vi "RemoveBus.vi"(7 "Remove All? (F)":bool, 8 "ErrorArray In":errorcluster[](array[cluster])) -> (0 "ErrorArray Out":errorcluster[](array[cluster]))   [LabVIEW 2017, in "Bus_class.lvlib" / "Bus.lvclass"]
uses:
  Bus.lvclass
  <userlib>/NIST/ModuleAdminLib/ModuleAdmin/ModuleAdmin.lvclass
  Bus.lvclass/Bus.ctl
  <vilib>/Utility/miscctls.llb/LVStringsAndValuesArrayTypeDef_U8.ctl
  Accessors/Read OutputToFileModuleID.vi
  <vilib>/Utility/error.llb/Error Cluster From Error Code.vi
  <vilib>/ErrorRing/Error Ring.xnode
  Modules/EventModule/EventModule.lvlib
  <userlib>/NIST/NISTErrorLib/NISTErrorLib.lvlib
  Framework.lvlib
  Modules/PmuImpairModule/PmuImpairModule.lvlib
  Modules/NetworkImpairmentModule/NetworkImpairmentModule.lvlib
  Modules/FlagImpairModule/FlagImpairModule.lvlib
  Bus_class.lvlib
  Modules/OutputToFileModule/OutputToFileModule.lvlib
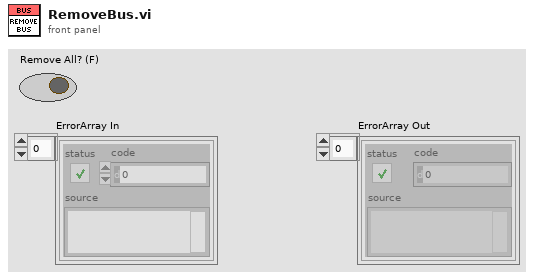
[diagram p1: front panel]
types:
  T1 = typedef "LVStringsAndValuesArrayTypeDef_U8.ctl" = cluster{"String":string, "Value":u8}[]
  T2 = typedef "Framework.lvlib/clFrontPanelControlRefs.ctl" = cluster{"TestFilePathRef":refnum<vi>, "BusNumberRef":refnum<vi>, "NumberOfBusesRef":refnum<vi>, "EvtTypeRef":refnum<vi>, "EvtParamsRef":refnum<vi>, "EvtConfigRef":refnum<vi>, "StartTimeRef":refnum<vi>, "EndTimeRef":refnum<vi>, "PmuImpairTypeRef":refnum<vi>, "PmuImpairParamsRef":refnum<vi>, "NetImpairParamsRef":refnum<vi>, "FlagImpairTypeRef":refnum<vi>, "FlagImpairParamsRef":refnum<vi>, "NetImpairTypeRef":refnum<vi>, "OutputFileType":refnum<vi>, "PmuImpairConfigRef":refnum<vi>, "AppTypeRef":refnum<vi>, "ScriptPathRef":refnum<vi>, "ShowPanels?":refnum<vi>}
  T3 = typedef "Framework.lvlib/clFrameworkData.ctl" = cluster{"EvtINIFilePaths":path[], "BusClassInstances":refnum<class "Bus.lvclass">[], "PmuImpairINIFilePaths":path[], "FlagImpairINIFilePaths":path[], "NetImpairINIFilePaths":path[], "OutputToFileINIFilePaths":path[], "AppINIFilePaths":path[], "AppModuleID":i32, "OutputToFileID":i32}
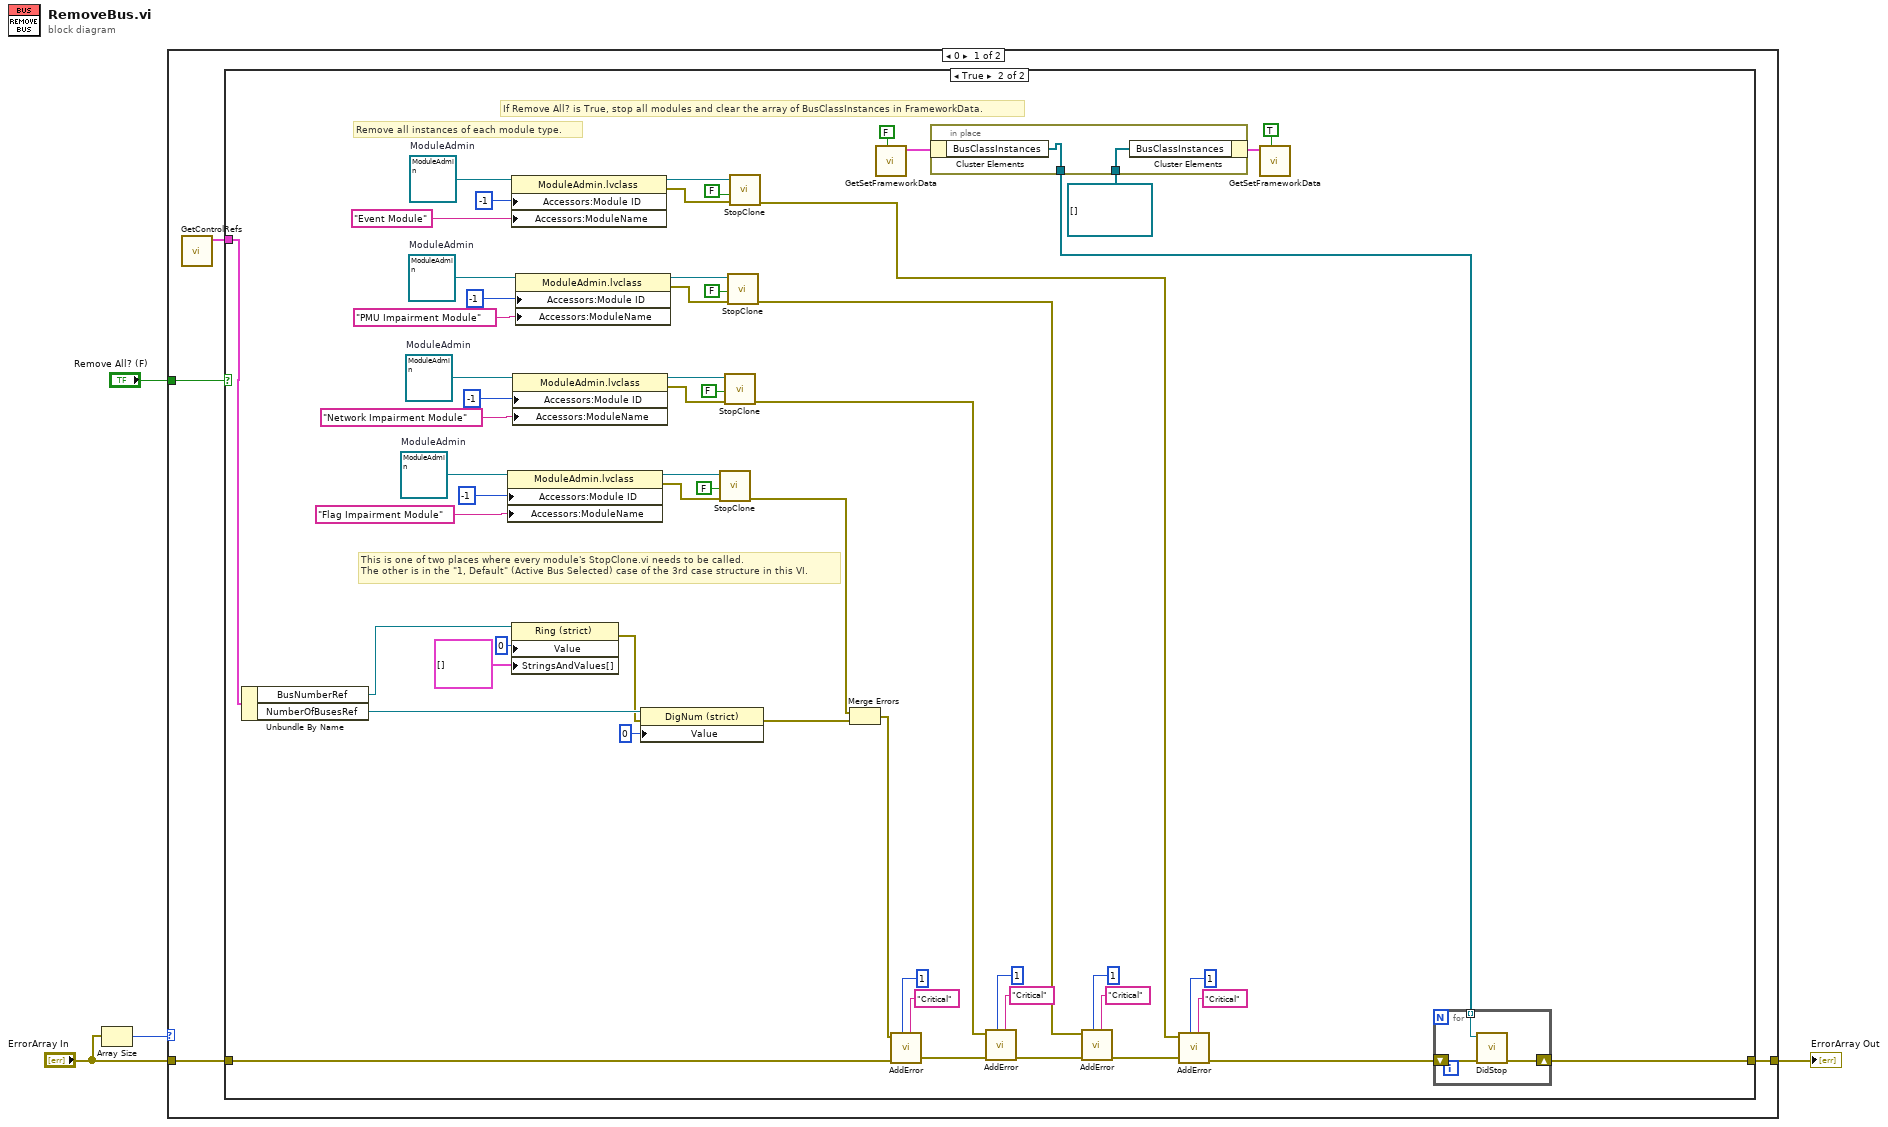
[diagram p0: block diagram]
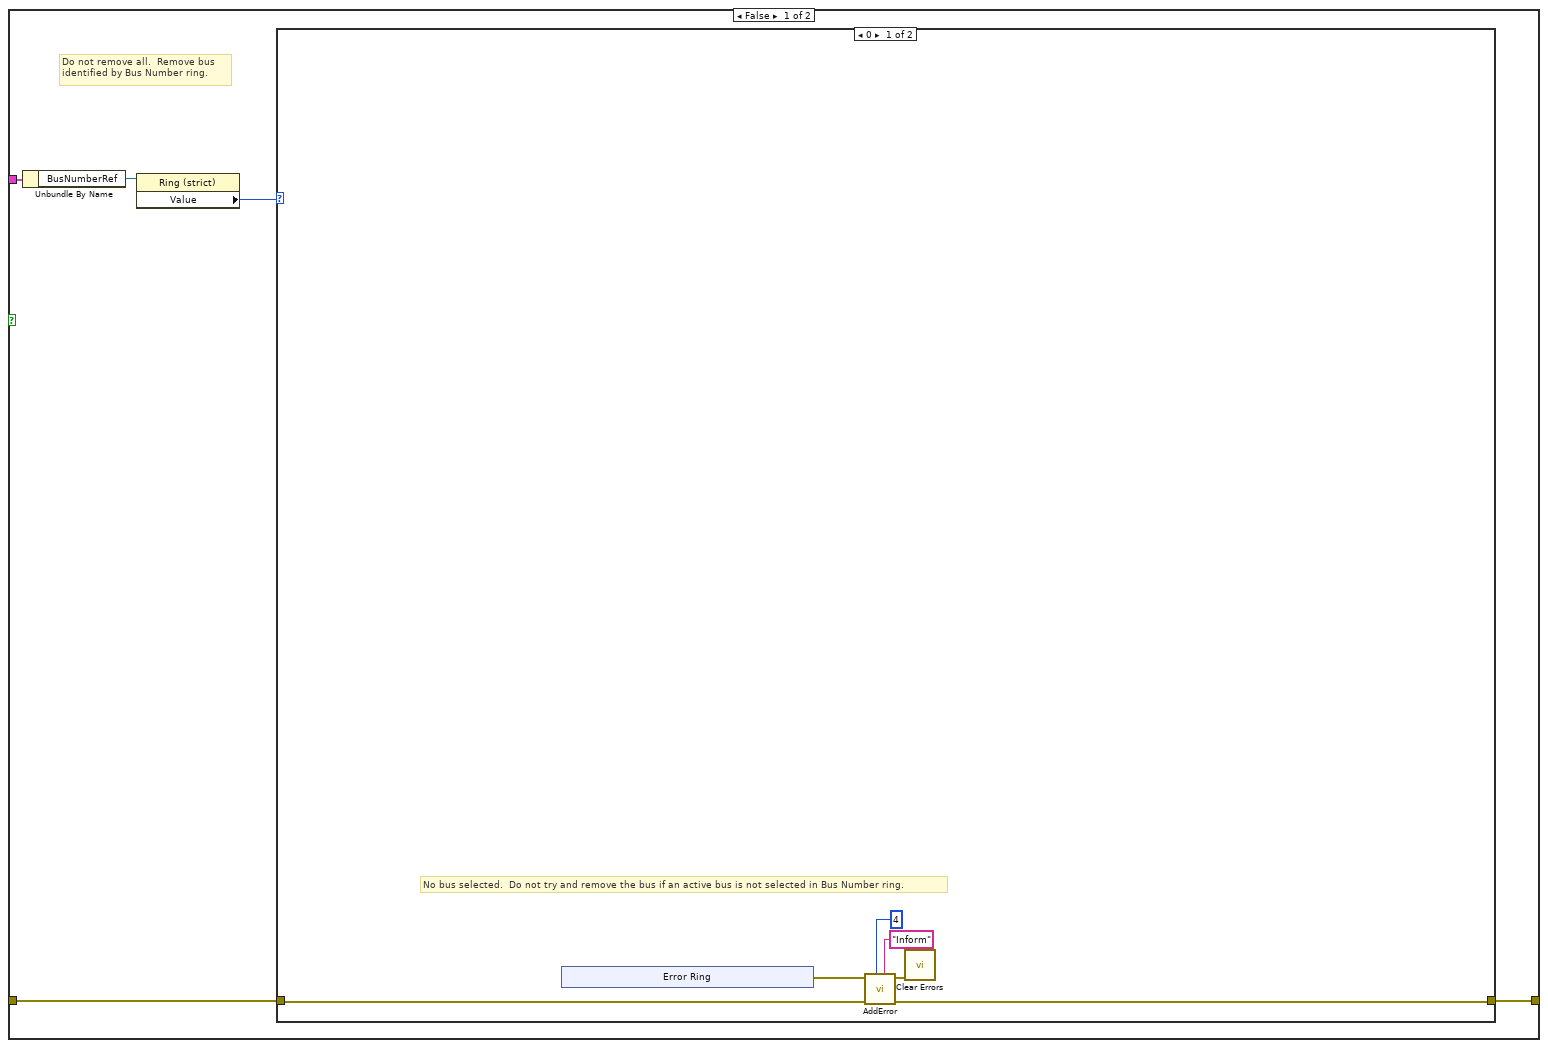
[diagram p2: hidden frame]
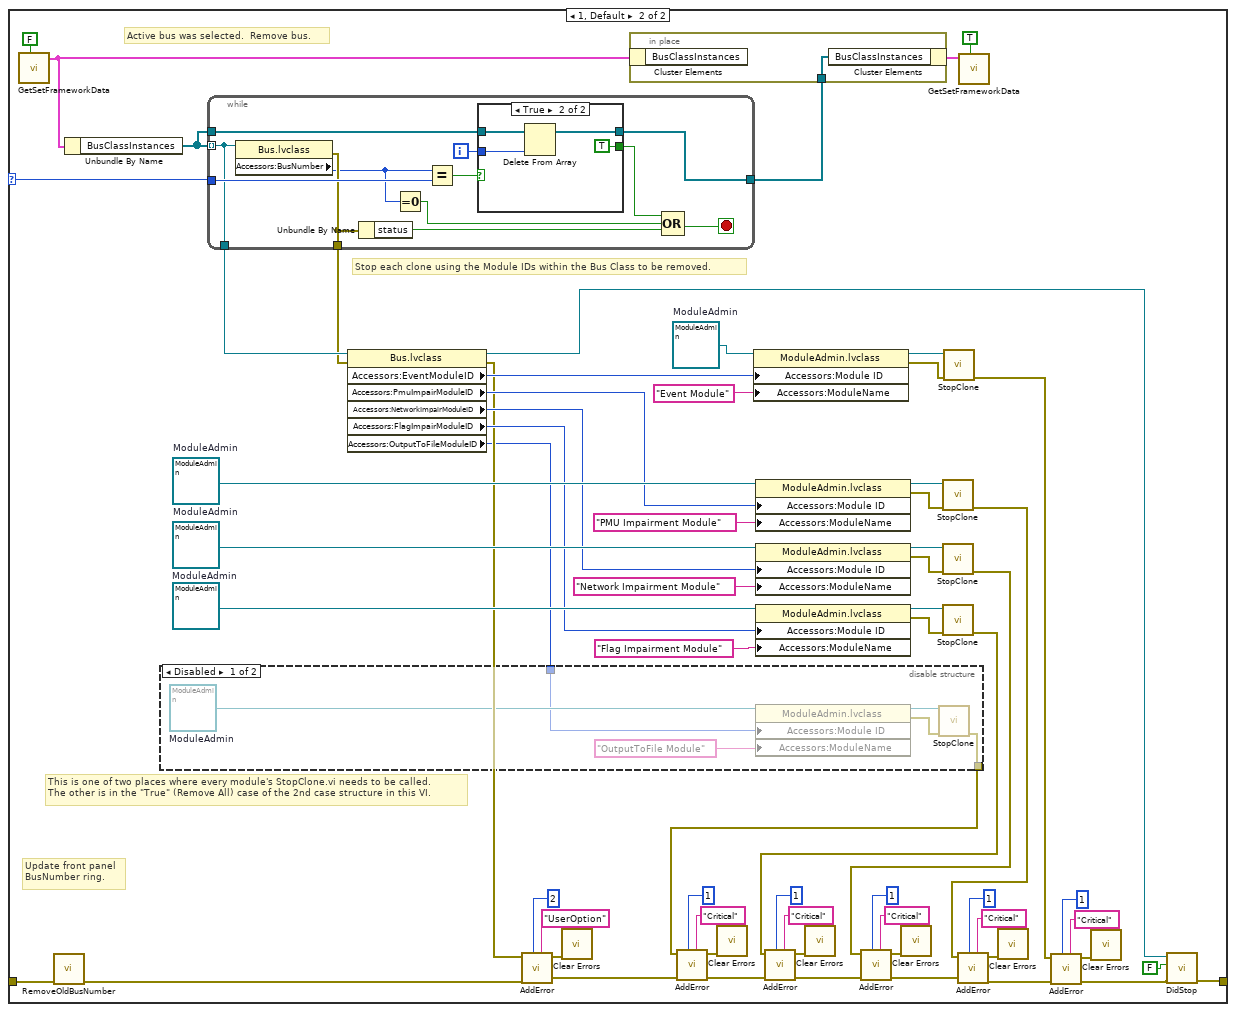
[diagram p3: hidden frame]
diagram:
  n1 = Array Size(array="ErrorArray In") -> (size(s)=w4:i32)
  n2 = case shown="0" w4 {
    tunnel: "ErrorArray In" -> [w7 w176]
    tunnel: [w8 w176] -> w2
    tunnel: "Remove All? (F)" -> [w6 _]
    frame 0 {
      n3 = call "GetControlRefs.vi"() -> ("clControlRefs Out"=w5:T2)  [unwired: 11 in]
      n4 = case shown="True" w6 {
        tunnel: [w13 w127] -> w8
        tunnel: w7 -> [w12 w124]
        tunnel: w5 -> [w9 w114]
        frame False {
          # "Do not remove all.  Remove bus\nidentified by Bus Number ring."
          n5 = Unbundle By Name(w9) -> ("BusNumberRef"=w11:refnum<vi>)
          n6 = property class="Ring (strict)"(reference=w11) -> ("Value"=w10:u8)  [unwired: 1 in, 2 out]
          n7 = case shown="0" w10 {
            selector: w10 -> [_ w77]
            tunnel: [w15 w34] -> w13
            tunnel: w12 -> [w16 w78]
            frame 0 {
              # "No bus selected.  Do not try and remove the bus if an active bus is not selected in Bus Number ring."
              n8 = xnode "Error Ring"() -> ("error out"=w14:errorcluster)
              n9 = call <userlib>:"AddError.vi"("Severity"="Inform" ("String"), "Priority"=u8 4, "ErrorArray"=w16, "error in (no error)"=w14) -> ("ErrorArray"=w15:errorcluster[], "error out"=w19:errorcluster)  [unwired: 6 in]
              n10 = call <vilib>:"Clear Errors.vi"("error in (no error)"=w19) -> ()  [unwired: 5 in, 2 out]
            }
            frame 1, Default {
              w59 = refnum<class "ModuleAdmin.lvclass"> refnum  # ModuleAdmin
              w65 = refnum<class "ModuleAdmin.lvclass"> refnum  # ModuleAdmin
              w69 = refnum<class "ModuleAdmin.lvclass"> refnum  # ModuleAdmin
              w72 = refnum<class "ModuleAdmin.lvclass"> refnum  # ModuleAdmin
              # "Update front panel\nBusNumber ring."
              # "This is one of two places where every module's StopClone.vi needs to be called.\nThe other is in the \"True\" (Remove All) case of the 2nd case structure in this VI."
              # "Stop each clone using the Module IDs within the Bus Class to be removed."
              # "Active bus was selected.  Remove bus."
              n11 = call "GetSetFrameworkData.vi"("Set (F)"=FALSE ("Set/Get")) -> ("clFrameworkData Out"=w85:T3)  [unwired: 10 in]
              n12 = call "RemoveOldBusNumber.vi"("ErrorArray In"=w78) -> ("ErrorArray Out"=w41:errorcluster[])  [unwired: 10 in]
              n13 = Unbundle By Name(w85) -> ("BusClassInstances"=w82:refnum<class "Bus.lvclass">[])
              n14 = while {
                tunnel: w77 -> [w106]
                tunnel: w82 -> [w102] mode=indexing
                tunnel: w82 -> [w105]
                tunnel: [w103] -> w81
                tunnel: [w102] -> w80
                tunnel: [w100] -> w79
                i -> [w104]
                stop <- w101 stop-if-true
                n15 = property class="Bus.lvclass"(reference=w102) -> (error out=w100:errorcluster, "Accessors:BusNumber"=w97:u8)  [unwired: 1 in, 1 out]
                n16 = Unbundle By Name(w100) -> ("status"=w99:bool)
                n17 = Equal To 0?(x=w97) -> (x = 0?=w96:bool)
                n18 = Equal?(x=w97, y=w106) -> (x = y?=w107:bool)
                n19 = case shown="True" w107 {
                  tunnel: w105 -> [w108 w112]
                  tunnel: w104 -> [_ w111]
                  tunnel: [_ TRUE] -> w98
                  tunnel: [w108 w109] -> w103
                  frame False {
                  }
                  frame True {
                    n20 = Delete From Array(array=w112, index=w111) -> (array with subset deleted=w109:refnum<class "Bus.lvclass">[])  [unwired: 1 in, 1 out]
                  }
                }
                n21 = Compound Arithmetic op=OR(w98, w96, w99) -> (w101:bool)
              }
              n22 = property class="Bus.lvclass"(reference=w80, error in=w79) -> (reference out=w33:refnum<class "Bus.lvclass">, error out=w40:errorcluster, "Accessors:EventModuleID"=w75:i32, "Accessors:PmuImpairModuleID"=w68:i32, "Accessors:NetworkImpairModuleID"=w62:i32, "Accessors:FlagImpairModuleID"=w57:i32, "Accessors:OutputToFileModuleID"=w31:i32)
              n23 = disable-structure shown="Disabled" {
                disable-tunnel: w31 -> [w93 _]
                disable-tunnel: [w90 _] -> w26
                frame Disabled {
                  w95 = refnum<class "ModuleAdmin.lvclass"> refnum  # ModuleAdmin
                  n24 = property class="ModuleAdmin.lvclass"(reference=w95, "Accessors:Module ID"=w93, "Accessors:ModuleName"="OutputToFile Module" ("ModuleName")) -> (reference out=w92:refnum<class "ModuleAdmin.lvclass">, error out=w91:errorcluster)  [unwired: 1 in]
                  n25 = call "StopClone.vi"("error in (no error)"=w91, "ModuleAdmin"=w92) -> ("error out"=w90:errorcluster)  [unwired: 9 in]
                }
                frame Enabled {
                }
              }
              n26 = call <userlib>:"AddError.vi"("Severity"="UserOption" ("String"), "Priority"=u8 2, "ErrorArray"=w41, "error in (no error)"=w40) -> ("ErrorArray"=w28:errorcluster[], "error out"=w45:errorcluster)  [unwired: 6 in]
              n27 = call <vilib>:"Clear Errors.vi"("error in (no error)"=w45) -> ()  [unwired: 5 in, 2 out]
              n28 = in-place {
                in-place-border: w81 -> [w113]
                n29 = in-place-cluster #1(w85) -> ()  [unwired: 1 out]
                n30 = in-place-cluster #1("BusClassInstances"=w113) -> (w83:T3)
              }
              n31 = call <userlib>:"AddError.vi"("Severity"="Critical" ("String"), "Priority"=u8 1, "ErrorArray"=w28, "error in (no error)"=w26) -> ("ErrorArray"=w27:errorcluster[], "error out"=w29:errorcluster)  [unwired: 6 in]
              n32 = call <vilib>:"Clear Errors.vi"("error in (no error)"=w29) -> ()  [unwired: 5 in, 2 out]
              n33 = property class="ModuleAdmin.lvclass"(reference=w72, "Accessors:Module ID"=w75, "Accessors:ModuleName"="Event Module") -> (reference out=w76:refnum<class "ModuleAdmin.lvclass">, error out=w73:errorcluster)  [unwired: 1 in]
              n34 = property class="ModuleAdmin.lvclass"(reference=w69, "Accessors:Module ID"=w68, "Accessors:ModuleName"="PMU Impairment Module") -> (reference out=w71:refnum<class "ModuleAdmin.lvclass">, error out=w70:errorcluster)  [unwired: 1 in]
              n35 = property class="ModuleAdmin.lvclass"(reference=w65, "Accessors:Module ID"=w62, "Accessors:ModuleName"="Network Impairment Module") -> (reference out=w63:refnum<class "ModuleAdmin.lvclass">, error out=w64:errorcluster)  [unwired: 1 in]
              n36 = property class="ModuleAdmin.lvclass"(reference=w59, "Accessors:Module ID"=w57, "Accessors:ModuleName"="Flag Impairment Module") -> (reference out=w61:refnum<class "ModuleAdmin.lvclass">, error out=w60:errorcluster)  [unwired: 1 in]
              n37 = call "StopClone.vi"("error in (no error)"=w70, "ModuleAdmin"=w71) -> ("error out"=w37:errorcluster)  [unwired: 9 in]
              n38 = call "StopClone.vi"("error in (no error)"=w64, "ModuleAdmin"=w63) -> ("error out"=w38:errorcluster)  [unwired: 9 in]
              n39 = call "StopClone.vi"("error in (no error)"=w60, "ModuleAdmin"=w61) -> ("error out"=w39:errorcluster)  [unwired: 9 in]
              n40 = call <userlib>:"AddError.vi"("Severity"="Critical" ("String"), "Priority"=u8 1, "ErrorArray"=w27, "error in (no error)"=w39) -> ("ErrorArray"=w44:errorcluster[], "error out"=w50:errorcluster)  [unwired: 6 in]
              n41 = call <vilib>:"Clear Errors.vi"("error in (no error)"=w50) -> ()  [unwired: 5 in, 2 out]
              n42 = call <userlib>:"AddError.vi"("Severity"="Critical" ("String"), "Priority"=u8 1, "ErrorArray"=w44, "error in (no error)"=w38) -> ("ErrorArray"=w43:errorcluster[], "error out"=w51:errorcluster)  [unwired: 6 in]
              n43 = call <vilib>:"Clear Errors.vi"("error in (no error)"=w51) -> ()  [unwired: 5 in, 2 out]
              n44 = call "StopClone.vi"("error in (no error)"=w73, "ModuleAdmin"=w76) -> ("error out"=w36:errorcluster)  [unwired: 9 in]
              n45 = call <userlib>:"AddError.vi"("Severity"="Critical" ("String"), "Priority"=u8 1, "ErrorArray"=w43, "error in (no error)"=w37) -> ("ErrorArray"=w42:errorcluster[], "error out"=w56:errorcluster)  [unwired: 6 in]
              n46 = call "GetSetFrameworkData.vi"("Set (F)"=TRUE ("Set/Get"), "clFrameworkData In"=w83) -> ()  [unwired: 9 in, 1 out]
              n47 = call <vilib>:"Clear Errors.vi"("error in (no error)"=w56) -> ()  [unwired: 5 in, 2 out]
              n48 = call <userlib>:"AddError.vi"("Severity"="Critical" ("String"), "Priority"=u8 1, "ErrorArray"=w42, "error in (no error)"=w36) -> ("ErrorArray"=w35:errorcluster[], "error out"=w89:errorcluster)  [unwired: 6 in]
              n49 = call <vilib>:"Clear Errors.vi"("error in (no error)"=w89) -> ()  [unwired: 5 in, 2 out]
              n50 = call "DidStop.vi"("ErrorArray"=w35, "Init?"=FALSE, "Bus"=w33) -> ("ErrorArray"=w34:errorcluster[])  [unwired: 7 in, 1 out]
            }
          }
        }
        frame True {
          w143 = refnum<class "ModuleAdmin.lvclass"> refnum  # ModuleAdmin
          w148 = refnum<class "ModuleAdmin.lvclass"> refnum  # ModuleAdmin
          w155 = refnum<class "ModuleAdmin.lvclass"> refnum  # ModuleAdmin
          w162 = refnum<class "ModuleAdmin.lvclass"> refnum  # ModuleAdmin
          # "This is one of two places where every module's StopClone.vi needs to be called.\nThe other is in the \"1, Default\" (Active Bus Selected) case of the 3rd case structure in this VI."
          # "Remove all instances of each module type."
          # "If Remove All? is True, stop all modules and clear the array of BusClassInstances in FrameworkData."
          n51 = Unbundle By Name(w114) -> ("BusNumberRef"=w123:refnum<vi>, "NumberOfBusesRef"=w122:refnum<vi>)
          n52 = property class="ModuleAdmin.lvclass"(reference=w143, "Accessors:Module ID"=-1 ("Module ID"), "Accessors:ModuleName"="Flag Impairment Module") -> (reference out=w145:refnum<class "ModuleAdmin.lvclass">, error out=w144:errorcluster)  [unwired: 1 in]
          n53 = property class="ModuleAdmin.lvclass"(reference=w162, "Accessors:Module ID"=-1 ("Module ID"), "Accessors:ModuleName"="Event Module") -> (reference out=w159:refnum<class "ModuleAdmin.lvclass">, error out=w158:errorcluster)  [unwired: 1 in]
          n54 = property class="Ring (strict)"(reference=w123, "Value"=u8 0, "StringsAndValues[]"=T1 [] ("Strings And Values []")) -> (error out=w120:errorcluster)  [unwired: 1 in, 1 out]
          n55 = property class="ModuleAdmin.lvclass"(reference=w148, "Accessors:Module ID"=-1 ("Module ID"), "Accessors:ModuleName"="Network Impairment Module") -> (reference out=w146:refnum<class "ModuleAdmin.lvclass">, error out=w147:errorcluster)  [unwired: 1 in]
          n56 = property class="ModuleAdmin.lvclass"(reference=w155, "Accessors:Module ID"=-1 ("Module ID"), "Accessors:ModuleName"="PMU Impairment Module") -> (reference out=w157:refnum<class "ModuleAdmin.lvclass">, error out=w156:errorcluster)  [unwired: 1 in]
          n57 = property class="DigNum (strict)"(reference=w122, error in=w120, "Value"=u8 0) -> (error out=w117:errorcluster)  [unwired: 1 out]
          n58 = call "StopClone.vi"("error in (no error)"=w144, "Wait for Module to stop?"=FALSE, "ModuleAdmin"=w145) -> ("error out"=w119:errorcluster)  [unwired: 8 in]
          n59 = call "StopClone.vi"("error in (no error)"=w147, "Wait for Module to stop?"=FALSE, "ModuleAdmin"=w146) -> ("error out"=w125:errorcluster)  [unwired: 8 in]
          n60 = call "StopClone.vi"("error in (no error)"=w156, "Wait for Module to stop?"=FALSE, "ModuleAdmin"=w157) -> ("error out"=w129:errorcluster)  [unwired: 8 in]
          n61 = call "StopClone.vi"("error in (no error)"=w158, "Wait for Module to stop?"=FALSE, "ModuleAdmin"=w159) -> ("error out"=w130:errorcluster)  [unwired: 8 in]
          n62 = Merge Errors(w119, w117) -> (w118:errorcluster)
          n63 = call "GetSetFrameworkData.vi"("Set (F)"=FALSE ("Set/Get")) -> ("clFrameworkData Out"=w169:T3)  [unwired: 10 in]
          n64 = call <userlib>:"AddError.vi"("Severity"="Critical" ("String"), "Priority"=u8 1, "ErrorArray"=w124, "error in (no error)"=w118) -> ("ErrorArray"=w133:errorcluster[])  [unwired: 6 in, 1 out]
          n65 = in-place {
            in-place-border: refnum<class "Bus.lvclass">[] [] ("BusClassInstances") -> [w175]
            in-place-border: [w174] -> w126
            n66 = in-place-cluster #2(w169) -> ("BusClassInstances"=w174:refnum<class "Bus.lvclass">[])
            n67 = in-place-cluster #2("BusClassInstances"=w175) -> (w167:T3)
          }
          n68 = call <userlib>:"AddError.vi"("Severity"="Critical" ("String"), "Priority"=u8 1, "ErrorArray"=w133, "error in (no error)"=w125) -> ("ErrorArray"=w132:errorcluster[])  [unwired: 6 in, 1 out]
          n69 = call <userlib>:"AddError.vi"("Severity"="Critical" ("String"), "Priority"=u8 1, "ErrorArray"=w132, "error in (no error)"=w129) -> ("ErrorArray"=w131:errorcluster[])  [unwired: 6 in, 1 out]
          n70 = call <userlib>:"AddError.vi"("Severity"="Critical" ("String"), "Priority"=u8 1, "ErrorArray"=w131, "error in (no error)"=w130) -> ("ErrorArray"=w128:errorcluster[])  [unwired: 6 in, 1 out]
          n71 = call "GetSetFrameworkData.vi"("Set (F)"=TRUE ("Set/Get"), "clFrameworkData In"=w167) -> ()  [unwired: 9 in, 1 out]
          n72 = for {
            shift-right: [w172] -> w127
            shift-left: w128 -> [w173]
            tunnel: w126 -> [w171] mode=indexing
            n73 = call "DidStop.vi"("ErrorArray"=w173, "Bus"=w171) -> ("ErrorArray"=w172:errorcluster[])  [unwired: 8 in, 1 out]
          }
        }
      }
    }
    frame 1, Default {
      # "External error.  Error array holds at least one error."
    }
  }
  "ErrorArray Out" <- w2
